vi "Calculation derivatives.vi"(8 "Save path 2":path=path "J:/20160720 陈老师 谷粒 米粒实验/binary&分割图/提取数据/谷粒米粒综合 +计算平均反射率.txt", 9 "Save path":path=path "J:/20160720 陈老师 谷粒 米粒实验/binary&分割图/提取数据/谷粒米粒综合 +计算平均反射率.txt", 11 "file path (dialog if empty)":path=path "J:/20160720 陈老师 谷粒 米粒实验/binary&分割图/提取数据/谷粒米粒综合 +计算平均反射率.txt") -> ()   [LabVIEW 2015]
uses:
  <vilib>/Utility/file.llb/Read Delimited Spreadsheet (string).vi
  <vilib>/Utility/file.llb/Write Delimited Spreadsheet (string).vi
  <vilib>/Analysis/NI_AALPro.lvlib
panel:
  out "output array 2":string[][](array[string])
  out "output array":string[][](array[string])
  out "all rows":string[][](array[string])
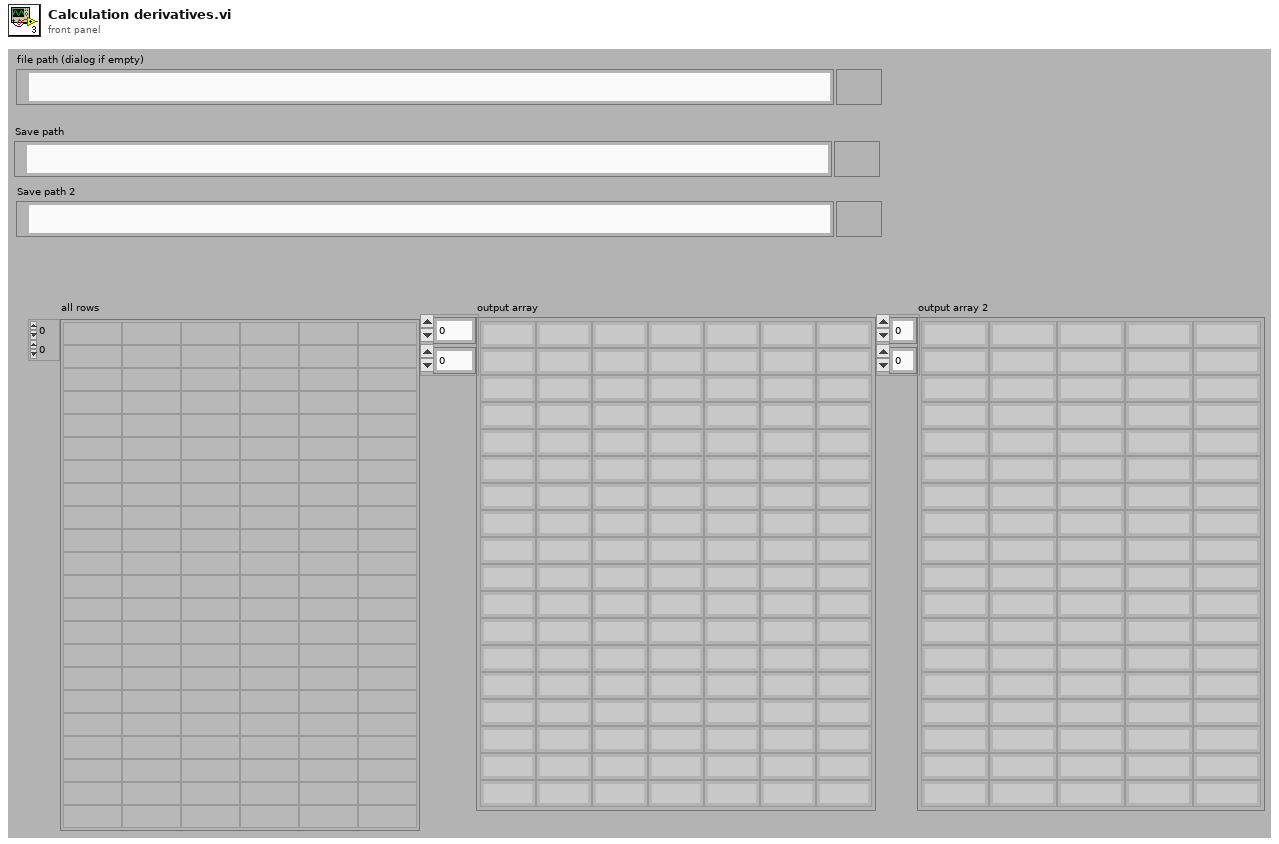
[diagram p1: front panel]
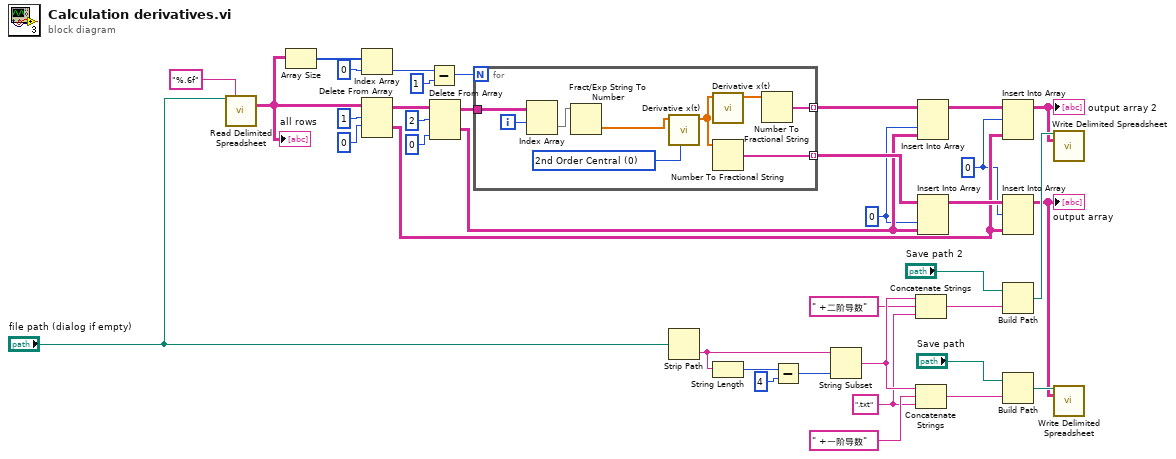
[diagram p0: block diagram]
diagram:
  w12 = 0 ("index")
  w8 = ".txt" ("string")
  w11 = 0 ("index (row)")
  n1 = call-poly <vilib>:"Read Delimited Spreadsheet.vi"("file path (dialog if empty)"="file path (dialog if empty)", "format (%s)"="%.6f" ("format (%.3f)")) -> ("all rows"=w5:string[][])  [unwired: 8 in, 5 out]
  "all rows" <- w5
  n2 = Array Size(array=w5) -> (size(s)=w37:i32[])
  n3 = Index Array(array=w37, index=0) -> (element=w19:i32)
  n4 = Delete From Array(array=w5, length=1, index (row)=0) -> (deleted portion=w13:string[][], array with subset deleted=w33:string[][])  [unwired: 1 in]
  n5 = Subtract(x=w19, y=1) -> (x-y=w23:i32)
  n6 = Delete From Array(array=w33, length=2, index (col)=0 ("index")) -> (deleted portion=w14:string[][], array with subset deleted=w20:string[][])  [unwired: 1 in]
  n7 = for {
    N: w23 -> [_]
    tunnel: [w47] -> w22 mode=indexing
    tunnel: w20 -> [w46]
    tunnel: [w39] -> w16 mode=indexing
    i -> [w44]
    w42 = u16 0 items=["2nd Order Central", "4th Order Central", "Forward", "Backward"] ("method")
    n8 = Index Array(array=w46, index (row)=w44) -> (element=w45:string[])  [unwired: 1 in]
    n9 = Fract/Exp String To Number(string=w45) -> (number=w43:dbl[])  [unwired: 4 out]
    n10 = call <vilib>:"Derivative x(t).vi"("method"=w42, "X"=w43) -> ("dX/dt"=w41:dbl[])  [unwired: 3 in, 6 out]
    n11 = call <vilib>:"Derivative x(t).vi"("X"=w41) -> ("dX/dt"=w40:dbl[])  [unwired: 4 in, 6 out]
    n12 = Number To Fractional String(number=w41) -> (F-format string=w47:string[])  [unwired: 3 out]
    n13 = Number To Fractional String(number=w40) -> (F-format string=w39:string[])  [unwired: 3 out]
  }
  n14 = Strip Path(path="file path (dialog if empty)") -> (name=w31:string)  [unwired: 1 out]
  n15 = String Length(string=w31) -> (length=w30:i32)
  n16 = Subtract(x=w30, y=4) -> (x-y=w28:i32)
  n17 = String Subset(string=w31, length (rest)=w28) -> (substring=w10:string)  [unwired: 1 out]
  n18 = Concatenate Strings(w10, " +二阶导数" ("string"), w8) -> (w7:string)
  n19 = Concatenate Strings(w10, " +一阶导数" ("string"), w8) -> (w27:string)
  n20 = Insert Into Array(array=w16, index (col)=w12, new element=w14) -> (w15:string[][])  [unwired: 1 in]
  n21 = Insert Into Array(array=w22, index (col)=w12, new element=w14) -> (w17:string[][])  [unwired: 1 in]
  n22 = Insert Into Array(array=w15, index (row)=w11, new element=w13) -> (w4:string[][])  [unwired: 1 in]
  "output array 2" <- w4
  n23 = Insert Into Array(array=w17, index (row)=w11, new element=w13) -> (w3:string[][])  [unwired: 1 in]
  "output array" <- w3
  n24 = Build Path(base path="Save path 2", name or relative path=w7) -> (appended path=w6:path)
  n25 = Build Path(base path="Save path", name or relative path=w27) -> (appended path=w25:path)
  n26 = call-poly <vilib>:"Write Delimited Spreadsheet.vi"("file path (dialog if empty)"=w6, "2D data"=w4) -> ()  [unwired: 12 in, 2 out]
  n27 = call-poly <vilib>:"Write Delimited Spreadsheet.vi"("file path (dialog if empty)"=w25, "2D data"=w3) -> ()  [unwired: 12 in, 2 out]
